vi "Get Status.vi"(11 "Framework in":refnum<class "Framework.lvclass">) -> (2 "Status":refnum<class "Framework Status.lvclass">, 3 "Framework out":refnum<class "Framework.lvclass">)   [LabVIEW 2017, in "Data Sharing Framework Core.lvlib" / "Data Sharing Framework Engine.lvlib" / "Framework.lvclass"]
uses:
  Framework.lvclass
  Internal/Execution/Framework Status/Framework Status.lvclass
  Framework.lvclass/Framework.ctl
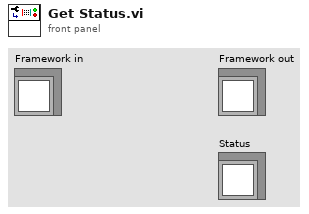
[diagram p1: front panel]
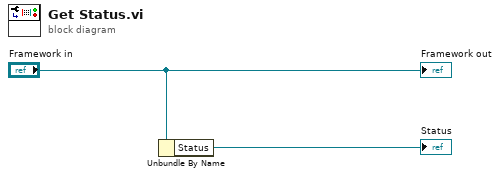
[diagram p0: block diagram]
diagram:
  n1 = Unbundle By Name("Framework in") -> ("Status"=→"Status":refnum<class "Framework Status.lvclass">)
  "Framework out" <- "Framework in"
